vi "备用系数写入.vi"(7 "备用系数":T1, 8 "error in (no error)":errorcluster, 9 "量程下拉列表":enum16{"低量程", "高量程"}(ring), 10 "测量模式":enum16{"跨度核查", "水样测量", "零点核查", "标样核查", "加标回收"}(ring), 11 "参数下拉列表":u16(ring) items=["总磷"=1, "总氮"=2]) -> (0 "error out":errorcluster)   [LabVIEW 2016, in "斯坦道总氮V2.lvlib"]
uses:
  <vilib>/Utility/error.llb/Error Cluster From Error Code.vi
  <vilib>/ErrorRing/Error Ring.xnode
  <vilib>/Plasmionique/MB Master/MB Master.lvlib
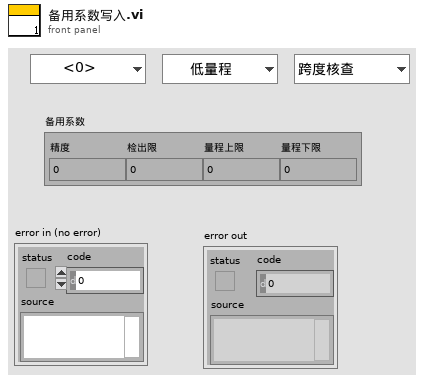
[diagram p1: front panel]
types:
  T1 = cluster{"精度":dbl, "检出限":dbl, "量程上限":dbl, "量程下限":dbl}
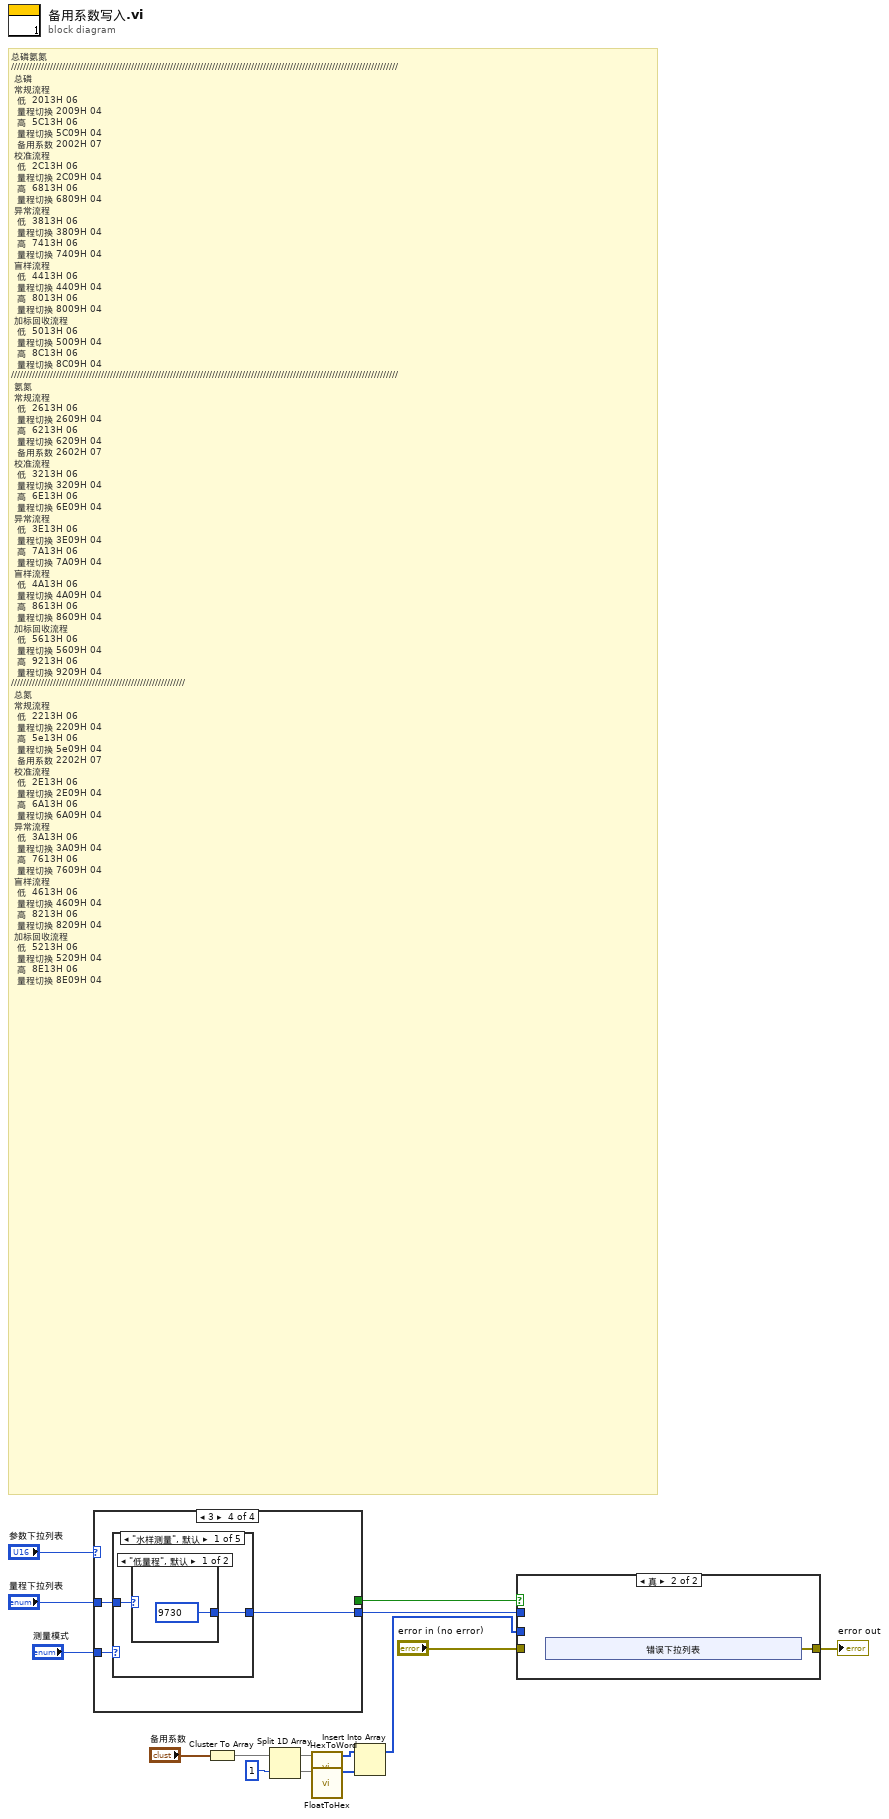
[diagram p0: block diagram]
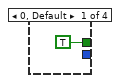
[diagram p2: hidden frame]
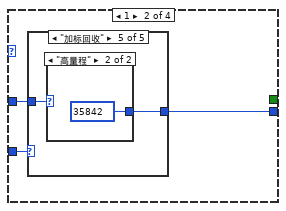
[diagram p3: hidden frame]
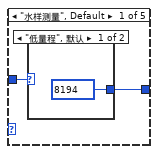
[diagram p4: hidden frame]
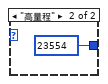
[diagram p5: hidden frame]
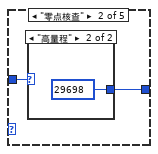
[diagram p6: hidden frame]
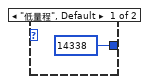
[diagram p7: hidden frame]
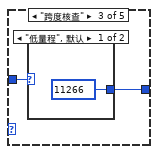
[diagram p8: hidden frame]
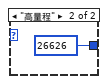
[diagram p9: hidden frame]
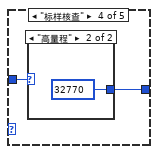
[diagram p10: hidden frame]
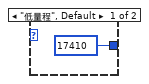
[diagram p11: hidden frame]
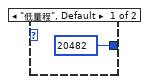
[diagram p12: hidden frame]
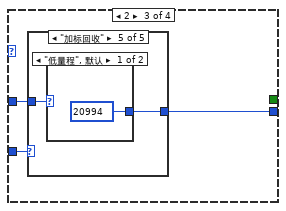
[diagram p13: hidden frame]
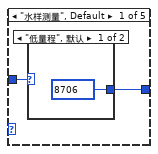
[diagram p14: hidden frame]
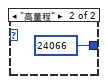
[diagram p15: hidden frame]
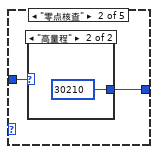
[diagram p16: hidden frame]
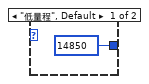
[diagram p17: hidden frame]
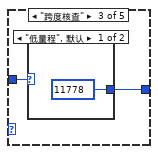
[diagram p18: hidden frame]
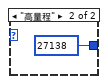
[diagram p19: hidden frame]
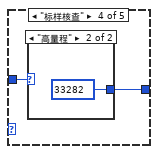
[diagram p20: hidden frame]
diagram:
  # "总磷氨氮\n/////////////////////////////////////////////////////////////////////////////////////////////////////////////////////////////////\n\t总磷\n\t常规流程\n\t\t低\t\t2013H\t06\n\t\t量程切换\t2009H\t04\n\t\t高\t\t5C13H\t06\n\t\t量程切换\t5C09H\t04\n\t\t备用系数\t2002H\t07\n\t校准流程\n\t\t低\t\t2C13H\t06\n\t\t量程切换\t2C09H\t04\n\t\t高\t\t6813H\t06\n\t\t量程切换\t6809H\t04\n\t异常流程\n\t\t低\t\t3813H\t06\n\t\t量程切换\t3809H\t04\n\t\t高\t\t7413H\t06\n\t\t量程切换\t7409H\t04\t\n\t盲样流程\n\t\t低\t\t4413H\t06\n\t\t量程切换\t4409H\t04\n\t\t高\t\t8013H\t06\n\t\t量程切换\t8009H\t04\t\n\t加标回收流程\n\t\t低\t\t5013H\t06\n\t\t量程切换\t5009H\t04\n\t\t高\t\t8C13H\t06\n\t\t量程切换\t8C09H\t04\t\n/////////////////////////////////////////////////////////////////////////////////////////////////////////////////////////////////\n\t氨氮\n\t常规流程\n\t\t低\t\t2613H\t06\n\t\t量程切换\t2609H\t04\n\t\t高\t\t6213H\t06\n\t\t量程切换\t6209H\t04\n\t\t备用系数\t2602H\t07\n\t校准流程\n\t\t低\t\t3213H\t06\n\t\t量程切换\t3209H\t04\n\t\t高\t\t6E13H\t06\n\t\t量程切换\t6E09H\t04\n\t异常流程\n\t\t低\t\t3E13H\t06\n\t\t量程切换\t3E09H\t04\n\t\t高\t\t7A13H\t06\n\t\t量程切换\t7A09H\t04\t\n\t盲样流程\n\t\t低\t\t4A13H\t06\n\t\t量程切换\t4A09H\t04\n\t\t高\t\t8613H\t06\n\t\t量程切换\t8609H\t04\t\n\t加标回收流程\n\t\t低\t\t5613H\t06\n\t\t量程切换\t5609H\t04\n\t\t高\t\t9213H\t06\n\t\t量程切换\t9209H\t04\t\n//////////////////////////////////////////////////////////\n\t总氮\n\t常规流程\n\t\t低\t\t2213H\t06\n\t\t量程切换\t2209H\t04\n\t\t高\t\t5e13H\t06\n\t\t量程切换\t5e09H\t04\n\t\t备用系数\t2202H\t07\n\t校准流程\n\t\t低\t\t2E13H\t06\n\t\t量程切换\t2E09H\t04\n\t\t高\t\t6A13H\t06\n\t\t量程切换\t6A09H\t04\n\t异常流程\n\t\t低\t\t3A13H\t06\n\t\t量程切换\t3A09H\t04\n\t\t高\t\t7613H\t06\n\t\t量程切换\t7609H\t04\t\n\t盲样流程\n\t\t低\t\t4613H\t06\n\t\t量程切换\t4609H\t04\n\t\t高\t\t8213H\t06\n\t\t量程切换\t8209H\t04\t\n\t加标回收流程\n\t\t低\t\t5213H\t06\n\t\t量程切换\t5209H\t04\n\t\t高\t\t8E13H\t06\n\t\t量程切换\t8E09H\t04"
  n1 = case shown="3" "参数下拉列表" {
    tunnel: "测量模式" -> [_ w19 w42 w65]
    tunnel: "量程下拉列表" -> [_ w18 w41 w64]
    tunnel: [_ w17 w40 w63] -> w9
    tunnel: [TRUE _ _ _] -> w8
    frame 0, Default {
    }
    frame 1 {
      n2 = case shown="\"加标回收\"" w19 {
        tunnel: w18 -> [w21 w25 w29 w33 w37]
        tunnel: [w20 w24 w28 w32 w36] -> w17
        frame "水样测量", Default {
          n3 = case shown="\"低量程\", 默认" w21 {
            tunnel: [u16 8194 ("starting address") u16 23554 ("starting address")] -> w20
            frame "低量程", Default {
            }
            frame "高量程" {
            }
          }
        }
        frame "零点核查" {
          n4 = case shown="\"高量程\"" w25 {
            tunnel: [u16 14338 ("starting address") u16 29698 ("starting address")] -> w24
            frame "低量程", Default {
            }
            frame "高量程" {
            }
          }
        }
        frame "跨度核查" {
          n5 = case shown="\"低量程\", 默认" w29 {
            tunnel: [u16 11266 ("starting address") u16 26626 ("starting address")] -> w28
            frame "低量程", Default {
            }
            frame "高量程" {
            }
          }
        }
        frame "标样核查" {
          n6 = case shown="\"高量程\"" w33 {
            tunnel: [u16 17410 ("starting address") u16 32770 ("starting address")] -> w32
            frame "低量程", Default {
            }
            frame "高量程" {
            }
          }
        }
        frame "加标回收" {
          n7 = case shown="\"高量程\"" w37 {
            tunnel: [u16 20482 ("starting address") u16 35842 ("starting address")] -> w36
            frame "低量程", Default {
            }
            frame "高量程" {
            }
          }
        }
      }
    }
    frame 2 {
      n8 = case shown="\"加标回收\"" w42 {
        tunnel: w41 -> [w44 w48 w52 w56 w60]
        tunnel: [w43 w47 w51 w55 w59] -> w40
        frame "水样测量", Default {
          n9 = case shown="\"低量程\", 默认" w44 {
            tunnel: [u16 8706 ("starting address") u16 24066 ("starting address")] -> w43
            frame "低量程", Default {
            }
            frame "高量程" {
            }
          }
        }
        frame "零点核查" {
          n10 = case shown="\"高量程\"" w48 {
            tunnel: [u16 14850 ("starting address") u16 30210 ("starting address")] -> w47
            frame "低量程", Default {
            }
            frame "高量程" {
            }
          }
        }
        frame "跨度核查" {
          n11 = case shown="\"低量程\", 默认" w52 {
            tunnel: [u16 11778 ("starting address") u16 27138 ("starting address")] -> w51
            frame "低量程", Default {
            }
            frame "高量程" {
            }
          }
        }
        frame "标样核查" {
          n12 = case shown="\"高量程\"" w56 {
            tunnel: [u16 17922 ("starting address") u16 33282 ("starting address")] -> w55
            frame "低量程", Default {
            }
            frame "高量程" {
            }
          }
        }
        frame "加标回收" {
          n13 = case shown="\"低量程\", 默认" w60 {
            tunnel: [u16 20994 ("starting address") u16 36354 ("starting address")] -> w59
            frame "低量程", Default {
            }
            frame "高量程" {
            }
          }
        }
      }
    }
    frame 3 {
      n14 = case shown="\"水样测量\", 默认" w65 {
        tunnel: w64 -> [w67 w71 w75 w79 w83]
        tunnel: [w66 w70 w74 w78 w82] -> w63
        frame "水样测量", Default {
          n15 = case shown="\"低量程\", 默认" w67 {
            tunnel: [u16 9730 ("starting address") u16 25090 ("starting address")] -> w66
            frame "低量程", Default {
            }
            frame "高量程" {
            }
          }
        }
        frame "零点核查" {
          n16 = case shown="\"低量程\", 默认" w71 {
            tunnel: [u16 15874 ("starting address") u16 31234 ("starting address")] -> w70
            frame "低量程", Default {
            }
            frame "高量程" {
            }
          }
        }
        frame "跨度核查" {
          n17 = case shown="\"低量程\", 默认" w75 {
            tunnel: [u16 12802 ("starting address") u16 28162 ("starting address")] -> w74
            frame "低量程", Default {
            }
            frame "高量程" {
            }
          }
        }
        frame "标样核查" {
          n18 = case shown="\"高量程\"" w79 {
            tunnel: [u16 18946 ("starting address") u16 34306 ("starting address")] -> w78
            frame "低量程", Default {
            }
            frame "高量程" {
            }
          }
        }
        frame "加标回收" {
          n19 = case shown="\"高量程\"" w83 {
            tunnel: [u16 22018 ("starting address") u16 37378 ("starting address")] -> w82
            frame "低量程", Default {
            }
            frame "高量程" {
            }
          }
        }
      }
    }
  }
  n20 = Cluster To Array(cluster="备用系数") -> (array=w6:dbl[])
  n21 = Split 1D Array(array=w6, index=1 ("索引")) -> (first subarray=w5:dbl[], second subarray=w4:dbl[])
  n22 = call "HexToWord.vi"("数组"=w5) -> ("WORD"=w3:u16[])  [unwired: 10 in]
  n23 = call "FloatToHex.vi"("浮点数"=w4) -> ("DCBA整形输出"=w2:u16[])  [unwired: 10 in]
  n24 = Insert Into Array(array=w3, new element=w2) -> (w1:u16[])  [unwired: 1 in]
  n25 = case shown="真" w8 {
    tunnel: w9 -> [w90 _]
    tunnel: w1 -> [w89 _]
    tunnel: "error in (no error)" -> [w87 _]
    tunnel: [w86 w91] -> w14
    frame False {
      n26 = global read "VAR总磷总氮全局变量.vi" "MB session in"() -> (w88:refnum<class "MB_Master.lvclass">)
      n27 = call <vilib>:"Write Multiple Registers.vi"("error in (no error)"=w87, "values"=w89, "starting address"=w90, "MB session in"=w88) -> ("error out"=w86:errorcluster)  [unwired: 6 in, 1 out]
    }
    frame True {
      n28 = xnode "错误下拉列表"() -> ("错误输出"=w91:errorcluster)
    }
  }
  "error out" <- w14
